vi "Layer_Get Active Clusters.vi"(5 "Get active Data only?":bool, 6 "Shift?":bool, 7 "Offset":i32, 8 "error in":errorcluster, 9 "Active Data":variant, 10 "CTRL?":bool, 11 "Absolut Pointer":u32) -> (0 "error out":errorcluster, 1 "Active Data out":u32[](array[numeric]), 3 "Relative Indices []":u32[](array[numeric]))   [LabVIEW 2021, in "FakedArray.lvclass"]
uses:
  <resource>/plugins/NIIconEditor/Class/FakedArray/FakedArray.lvclass
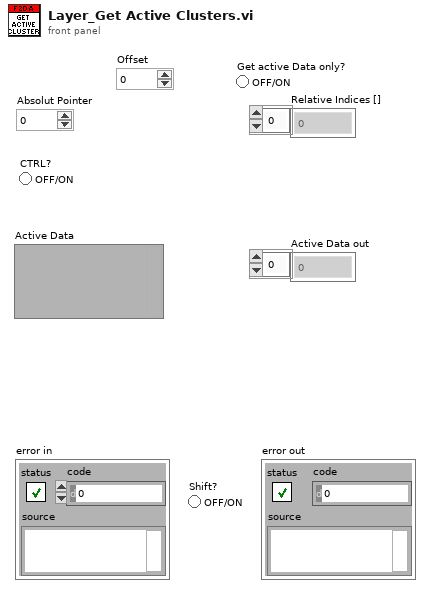
[diagram p1: front panel]
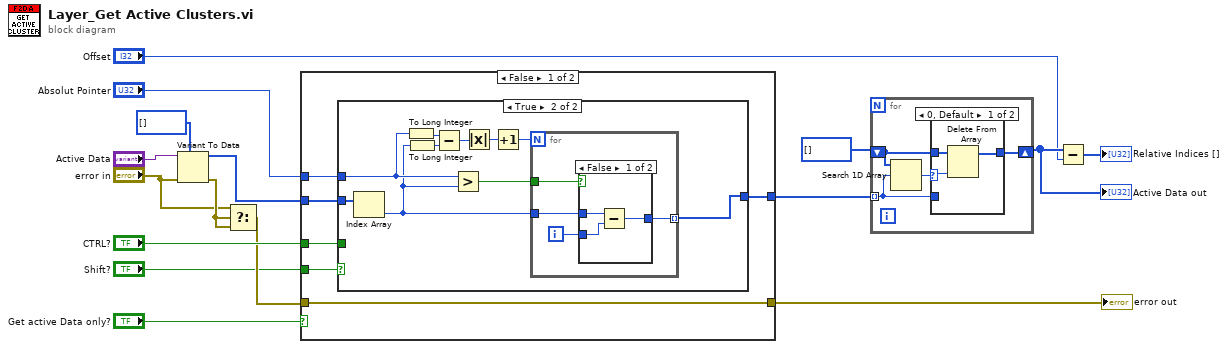
[diagram p0: block diagram]
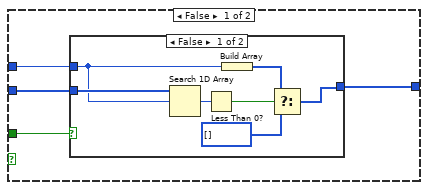
[diagram p2: hidden frame]
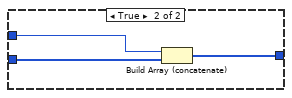
[diagram p3: hidden frame]
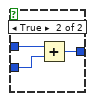
[diagram p4: hidden frame]
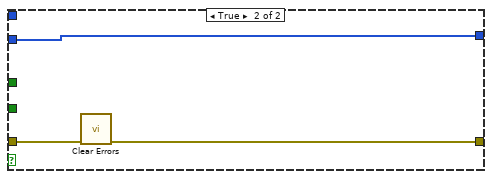
[diagram p5: hidden frame]
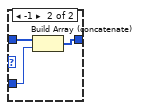
[diagram p6: hidden frame]
diagram:
  n1 = Variant To Data(error in="error in", type=u32[] [], Variant="Active Data") -> (data=w6:u32[], error out=w12:errorcluster)
  n2 = Select(t="error in", s=w12, f=w12) -> (s? t:f=w4:errorcluster)
  n3 = case shown="False" "Get active Data only?" {
    tunnel: [w22 w57] -> w14
    tunnel: "Absolut Pointer" -> [w21 _]
    tunnel: "CTRL?" -> [w20 _]
    tunnel: w6 -> [w19 w57]
    tunnel: w4 -> [w18 w59]
    tunnel: [w18 w58] -> w3
    tunnel: "Shift?" -> [w17 _]
    frame False {
      n4 = case shown="True" w17 {
        tunnel: [w26 w37] -> w22
        tunnel: w21 -> [w25 w39]
        tunnel: w20 -> [w24 _]
        tunnel: w19 -> [w23 w46]
        frame False {
          n5 = case shown="False" w24 {
            tunnel: w23 -> [w33 w36]
            tunnel: w25 -> [w30 w35]
            tunnel: [w28 w34] -> w26
            frame False {
              n6 = Search 1D Array(1D array=w33, element=w30) -> (index of element=w32:i32)  [unwired: 1 out]
              n7 = Less Than 0?(x=w32) -> (x < 0?=w31:bool)
              n8 = Build Array(w30) -> (w29:u32[])
              n9 = Select(t=w29, s=w31, f=u32[] []) -> (s? t:f=w28:u32[])
            }
            frame True {
              n10 = Build Array (concatenate)(w35, w36) -> (w34:u32[])
            }
          }
        }
        frame True {
          n11 = Index Array(array=w46) -> (element=w38:u32)  [unwired: 1 in]
          n12 = To Long Integer(number=w39) -> (32bit integer=w42:i32)
          n13 = To Long Integer(number=w38) -> (32bit integer=w44:i32)
          n14 = Subtract(x=w42, y=w44) -> (x-y=w43:i32)
          n15 = Greater?(x=w39, y=w38) -> (0:w41:bool)
          n16 = Absolute Value(x=w43) -> (abs(x)=w45:i32)
          n17 = Increment(x=w45) -> (x+1=w40:i32)
          n18 = for {
            N: w40 -> [_]
            tunnel: w41 -> [w50]
            tunnel: w38 -> [w49]
            tunnel: [w47] -> w37 mode=indexing
            i -> [w48]
            n19 = case shown="False" w50 {
              tunnel: w49 -> [w53 w56]
              tunnel: w48 -> [w52 w55]
              tunnel: [w51 w54] -> w47
              frame False {
                n20 = Subtract(x=w53, y=w52) -> (x-y=w51:u32)
              }
              frame True {
                n21 = Add(x=w56, y=w55) -> (x+y=w54:u32)
              }
            }
          }
        }
      }
    }
    frame True {
      n22 = call <vilib>:"Clear Errors.vi"("error in (no error)"=w59) -> ("error out"=w58:errorcluster)  [unwired: 1 in, 5 out]
    }
  }
  "error out" <- w3
  n23 = for {
    tunnel: w14 -> [w61] mode=indexing
    shift-right: [w60] -> w10
    shift-left: u32[] [] -> [w62]
    n24 = Search 1D Array(1D array=w62, element=w61) -> (index of element=w63:i32)  [unwired: 1 out]
    n25 = case shown="0, Default" w63 {
      selector: w63 -> [w65 _]
      tunnel: w62 -> [w66 w69]
      tunnel: w61 -> [_ w68]
      tunnel: [w64 w67] -> w60
      frame 0, Default {
        n26 = Delete From Array(array=w66, index=w65) -> (array with subset deleted=w64:u32[])  [unwired: 1 in, 1 out]
      }
      frame -1 {
        n27 = Build Array (concatenate)(w69, w68) -> (w67:u32[])
      }
    }
  }
  "Active Data out" <- w10
  n28 = Subtract(x=w10, y="Offset") -> (x-y=→"Relative Indices []":u32[])
